vi "niScope Configure Clock.vi"(0 "instrument handle":refnum<k15>, 1 "input clock source":T3 caption="reference (input) clock source" items=["None"=0, "RTSI Clock"=1, "PFI 0"=6, "PFI 1"=2, "PFI 2"=3, "PXI Clock"=4, "External"=5, "Clock In"=7], 5 "clock sync pulse source":T2=9 items=["RTSI 0", "RTSI 1", "RTSI 2", "RTSI 3", "RTSI 4", "RTSI 5", "RTSI 6", "PFI 1", "PFI 2", "Internal"], 9 "master enabled":bool=TRUE, 11 "error in":errorcluster, 12 "output clock source":T1 items=["None"=0, "PFI 0"=4, "PFI 1"=2, "PFI 2"=3, "RTSI 0"=5, "RTSI 1"=6, "RTSI 2"=7, "RTSI 3"=8, "RTSI 4"=9, "RTSI 5"=10, "RTSI 6"=11, "RTSI Clock"=1, "Clock Out"=12]) -> (4 "instrument handle out":refnum<k15>, 15 "error out":errorcluster)   [LabVIEW 2013]
doc: "Configures the properties for synchronizing the digitizer to an external clock or sending the digitizer's clock output to be used as a synchronizing clock for other devices."
uses:
  <instrlib>/niScope/Controls/niScope input clock source.ctl
  <instrlib>/niScope/Controls/niScope clock sync pulse source.ctl
  <instrlib>/niScope/Controls/niScope output clock source.ctl
  niScope_32.dll
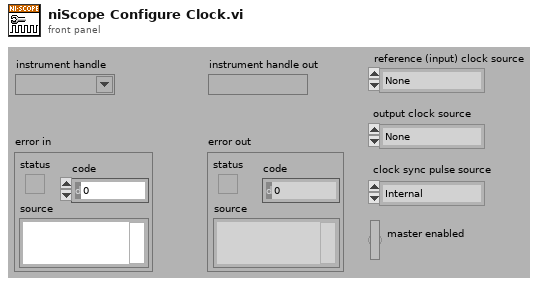
[diagram p1: front panel]
types:
  T1 = typedef "niScope output clock source.ctl" = u16
  T2 = typedef "niScope clock sync pulse source.ctl" = u16
  T3 = typedef "niScope input clock source.ctl" = u16
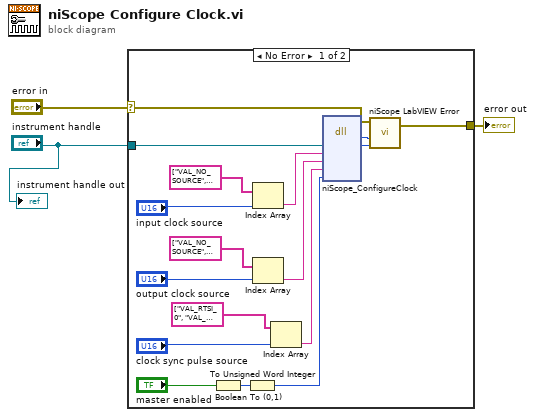
[diagram p0: block diagram]
diagram:
  n1 = case shown="No Error" "error in" {
    selector: "error in" -> [w5 w21]
    tunnel: [w6 w21] -> w3
    tunnel: "instrument handle" -> [w20 _]
    frame No Error {
      n2 = Boolean To (0,1)(Boolean="master enabled") -> (0, 1=w18:i16)
      n3 = To Unsigned Word Integer(number=w18) -> (unsigned 16bit integer=w11:u16)
      n4 = Index Array(array=string[] ["VAL_NO_SOURCE", "VAL_RTSI_CLOCK", "VAL_PFI_1", "VAL_PFI_2", "VAL_PXI_CLOCK", "VAL_EXTERNAL", "VAL_PFI_0", "VAL_CLK_IN"] ("input clock source array"), index="input clock source") -> (element=w16:string)
      n5 = Index Array(array=string[] ["VAL_NO_SOURCE", "VAL_RTSI_CLOCK", "VAL_PFI_1", "VAL_PFI_2", "VAL_PFI_0", "VAL_RTSI_0", "VAL_RTSI_1", "VAL_RTSI_2", "VAL_RTSI_3", "VAL_RTSI_4", "VAL_RTSI_5", "VAL_RTSI_6", "VAL_CLK_OUT"] ("output clock source array"), index="output clock source") -> (element=w15:string)
      n6 = Index Array(array=string[] ["VAL_RTSI_0", "VAL_RTSI_1", "VAL_RTSI_2", "VAL_RTSI_3", "VAL_RTSI_4", "VAL_RTSI_5", "VAL_RTSI_6", "VAL_PFI_1", "VAL_PFI_2", "VAL_NO_SOURCE"] ("clock sync pulse source array"), index="clock sync pulse source") -> (element=w12:string)
      n7 = dll-call lib="niScope_*.*" fn="niScope_ConfigureClock"("instrument handle"=w20, "inputClockSource"=w16, "outputClockSource"=w15, "clockSyncPulseSource"=w12, "masterEnabled"=w11) -> ("status"=w7:i32, "instrument handle"=w8:u32)  [unwired: 7 in, 2 out]
      n8 = call <instrlib>:"niScope LabVIEW Error.vi"("instrument handle"=w8, "niScope error code (0)"=w7, "error in (no error)"=w5) -> ("error out"=w6:errorcluster)  [unwired: 2 in]
    }
    frame Error {
    }
  }
  "error out" <- w3
  "instrument handle out" <- "instrument handle"
